vi "Write IncFreq.vi"(8 "error in (no error)":errorcluster, 10 "IncFreq":dbl, 11 "ChirpEIS in":refnum<class "ChirpEIS.lvclass">) -> (0 "error out":errorcluster, 3 "ChirpEIS out":refnum<class "ChirpEIS.lvclass">)   [LabVIEW 2014, in "ChirpEIS.lvclass"]
uses:
  ChirpEIS.lvclass
  ChirpEIS.lvclass/ChirpEIS.ctl
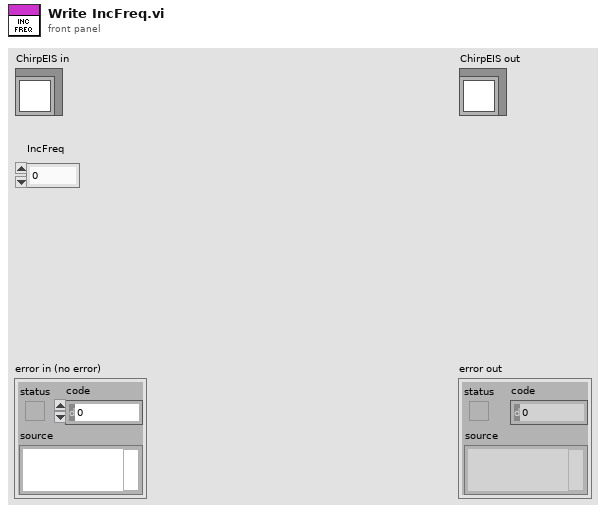
[diagram p1: front panel]
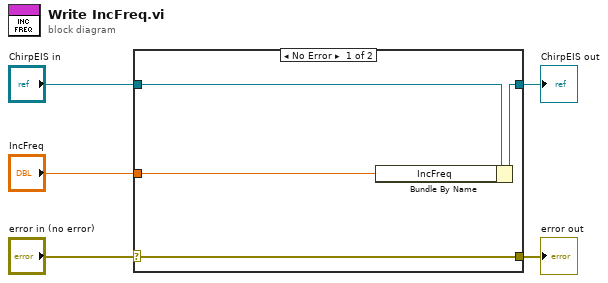
[diagram p0: block diagram]
diagram:
  n1 = case shown="No Error" "error in (no error)" {
    selector: "error in (no error)" -> [w9 w10]
    tunnel: [w9 w10] -> w4
    tunnel: [w7 w11] -> w2
    tunnel: "ChirpEIS in" -> [w8 w11]
    tunnel: "IncFreq" -> [w6 _]
    frame No Error {
      n2 = Bundle By Name(cluster=w8, "IncFreq"=w6) -> (w7:refnum<class "ChirpEIS.lvclass">)
    }
    frame Error {
    }
  }
  "error out" <- w4
  "ChirpEIS out" <- w2
